vi "Right Join.vi"() -> ()   [LabVIEW 2020]
uses:
  a75eeadb-a20a-426b-b48b-c9c06ab4b909.vi
  965599a9-35c5-4084-8906-0a043779e57e.vi
panel:
  out "array with duplicates removed":string[][](array[string])
  in  "Array 2":string[][](array[string])
  in  "Array":string[][](array[string])
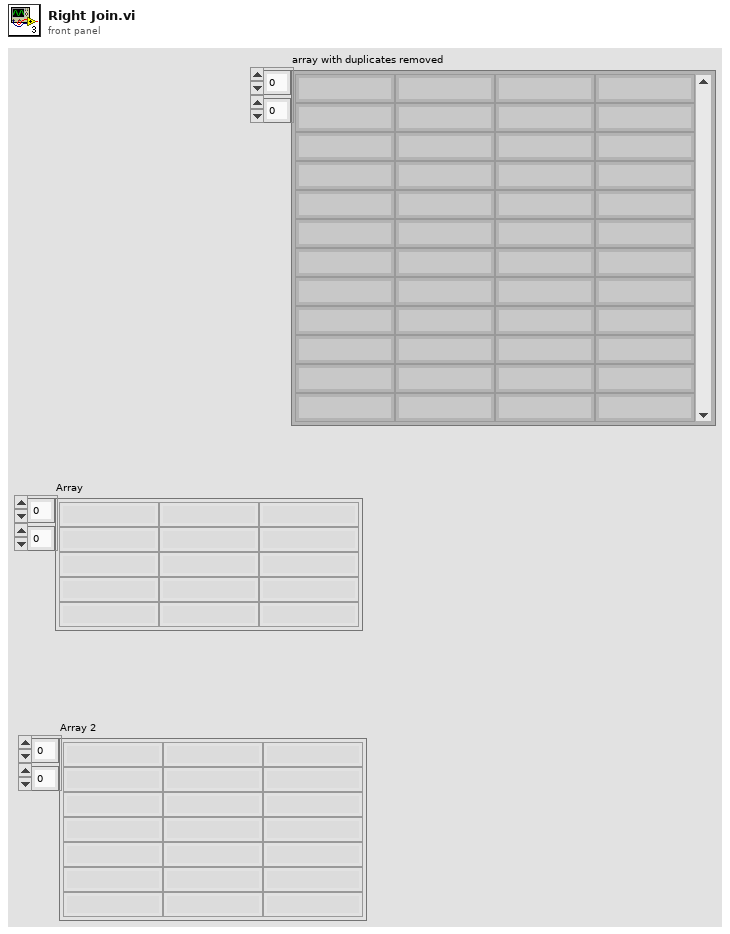
[diagram p1: front panel]
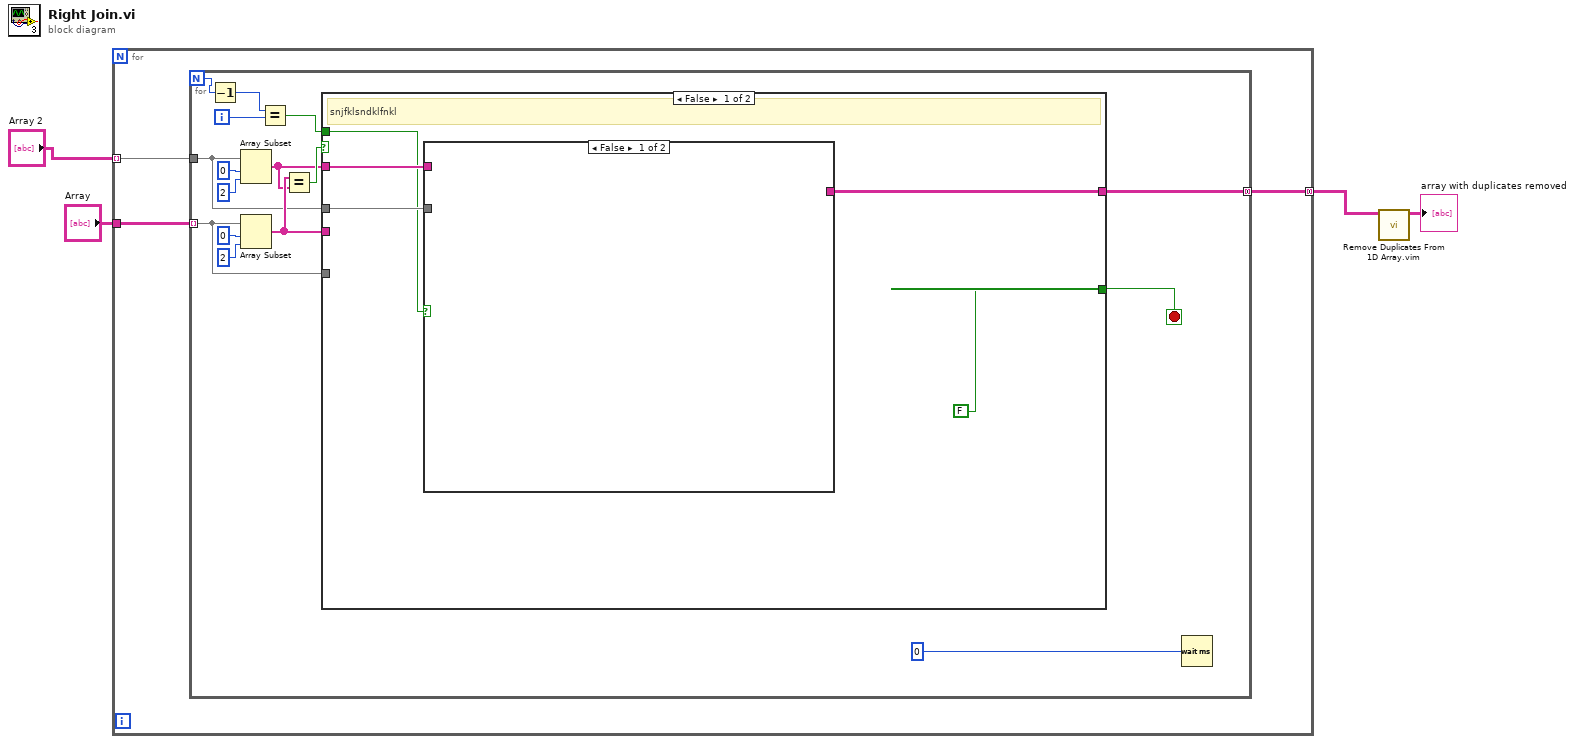
[diagram p0: block diagram]
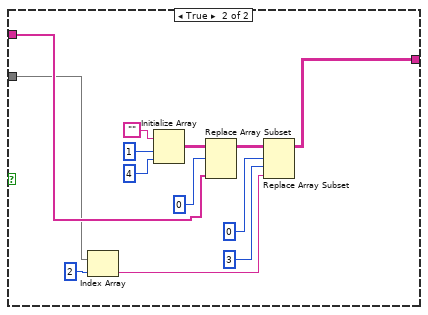
[diagram p2: hidden frame]
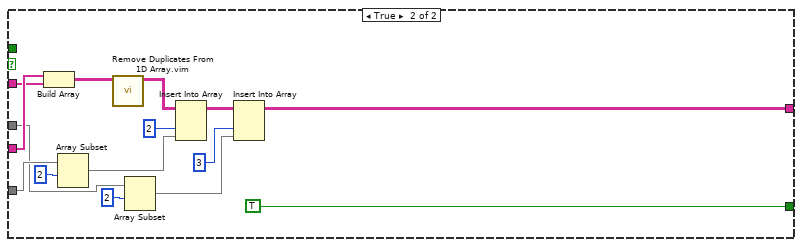
[diagram p3: hidden frame]
diagram:
  n1 = for {
    tunnel: "Array" -> [w6]
    tunnel: [w7] -> w3 mode=concatenating
    tunnel: "Array 2" -> [w5] mode=indexing
    n2 = for {
      N -> [w11]
      tunnel: w5 -> [w15]
      tunnel: w6 -> [w17] mode=indexing
      tunnel: [w22] -> w7 mode=concatenating
      i -> [w9]
      stop <- w12 stop-if-true
      n3 = Decrement(x=w11) -> (x-1=w10:i32)
      n4 = Array Subset(array=w15, index=0, length=2) -> (w14:string[])
      n5 = Array Subset(array=w17, index=0, length=2) -> (w16:string[])
      n6 = Equal?(x=w10, y=w9) -> (x = y?=w8:bool)
      n7 = Equal?(x=w16, y=w14) -> (x = y?=w23:bool)
      n8 = case shown="False" w23 {
        tunnel: [w28 w45] -> w22
        tunnel: w17 -> [_ w52]
        tunnel: w15 -> [w26 w49]
        tunnel: w16 -> [_ w56]
        tunnel: w14 -> [w27 w55]
        tunnel: [FALSE TRUE] -> w12
        tunnel: w8 -> [w24 _]
        frame False {
          # "snjfklsndklfnkl"
          n9 = case shown="False" w24 {
            tunnel: [_ w31] -> w28
            tunnel: w27 -> [_ w30]
            tunnel: w26 -> [_ w29]
            frame False {
            }
            frame True {
              n10 = Index Array(array=w29, index=2) -> (element=w38:string)
              n11 = Initialize Array("", 1 ("dimension size"), 4 ("dimension size")) -> (w34:string[][])
              n12 = Replace Array Subset(array=w34, new element=w30, index (row)=0) -> (w32:string[][])  [unwired: 1 in]
              n13 = Replace Array Subset(array=w32, new element=w38, index (row)=0 ("disabled index (row)"), index (col)=3 ("index (row)")) -> (w31:string[][])
            }
          }
        }
        frame True {
          n14 = Build Array(w56, w55) -> (w54:string[][])
          n15 = Array Subset(array=w52, index=2) -> (w51:string[])  [unwired: 1 in]
          n16 = call "Remove Duplicates From 1D Array.vim"("array"=w54) -> ("array with duplicates removed"=w53:string[][])  [unwired: 10 in]
          n17 = Array Subset(array=w49, index=2) -> (w46:string[])  [unwired: 1 in]
          n18 = Insert Into Array(array=w53, index (col)=2 ("index (row)"), new element=w51) -> (w47:string[][])  [unwired: 1 in]
          n19 = Insert Into Array(array=w47, index (col)=3 ("index (row)"), new element=w46) -> (w45:string[][])  [unwired: 1 in]
        }
      }
      n20 = Wait (ms)(milliseconds to wait=u32 0) -> ()  [unwired: 1 out]
    }
  }
  n21 = call "Remove Duplicates From 1D Array.vim"("array"=w3) -> ("array with duplicates removed"=→"array with duplicates removed":string[][])  [unwired: 10 in]
